vi "nanonocal_temperature_calibration_manage_V1.vi"(6 "calibartion table file path":path, 7 "calibration table action":T1, 10 "R (Ohm)":dbl format="%#_13g") -> (0 "dT/dR OUT (K/Ohm)":dbl format="%#_13g", 1 "T OUT (K)":dbl format="%#_13g", 2 "R OUT (Ohm)":dbl format="%#_13g")   [LabVIEW 2021]
uses:
  nanocal_calibration_table_actionV1.ctl
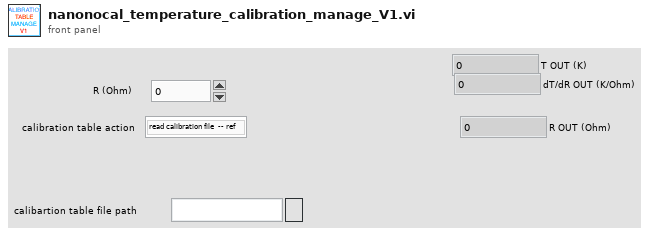
[diagram p1: front panel]
types:
  T1 = typedef "nanocal_calibration_table_actionV1.ctl" = enum16{"read calibration file  -- ref", "read calibration file  -- sam", "calc dTr/dRr", "calc dTs/dRs"}
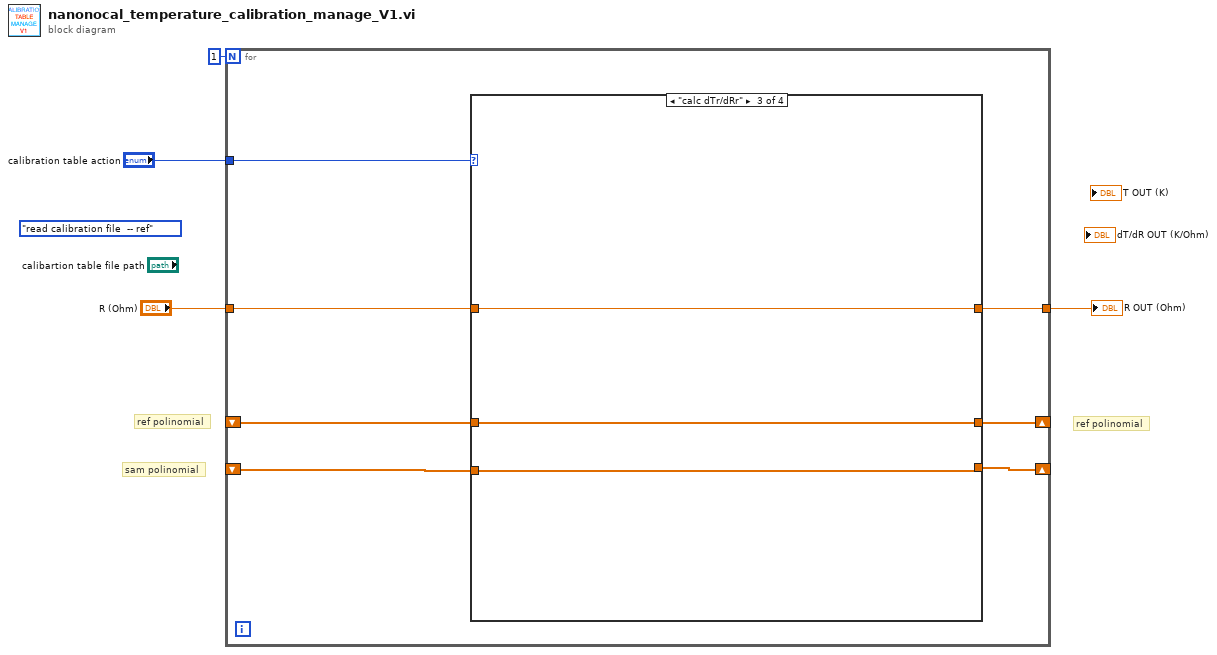
[diagram p0: block diagram]
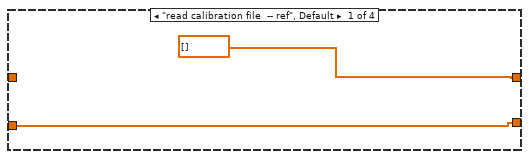
[diagram p2: hidden frame]
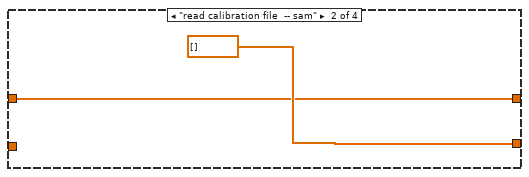
[diagram p3: hidden frame]
diagram:
  (unwired) nanocal_calibration_table_actionV1."read calibration file  -- ref" ("calibration table action")
  # "ref polinomial"
  # "sam polinomial"
  # "ref polinomial"
  n1 = for {
    N: 1 -> [_]
    shift-right: [w10] -> _
    shift-left: _ -> [w8]
    tunnel: "calibration table action" -> [w11]
    shift-right: [w9] -> _
    shift-left: _ -> [w7]
    tunnel: "R (Ohm)" -> [w6]
    tunnel: [w5] -> w1
    n2 = case shown="\"calc dTr/dRr\"" w11 {
      tunnel: [dbl[] [] w14 w17 _] -> w10
      tunnel: [w12 dbl[] [] w18 _] -> w9
      tunnel: w8 -> [_ w14 w17 _]
      tunnel: w7 -> [w12 _ w18 _]
      tunnel: w6 -> [_ _ w16 _]
      tunnel: [_ _ w16 _] -> w5
      frame "read calibration file  -- ref", Default {
      }
      frame "read calibration file  -- sam" {
      }
      frame "calc dTr/dRr" {
      }
      frame "calc dTs/dRs" {
      }
    }
  }
  "R OUT (Ohm)" <- w1
